vi "Training-Master-Slave.vi"() -> ()   [LabVIEW 2016]
doc: "Use this template to build a master/slave design pattern. The master loop always executes. It notifies one or more slave loops to execute their code. The slave loop(s) continue executing until they complete, then wait for another notification. Contrast this with the Producer/Consumer pattern in which the consumer loops execute only when they have data in their queue."
panel:
  out "notification":dbl[](array[numeric])
  in  "Device":u32
  in  "stop":bool
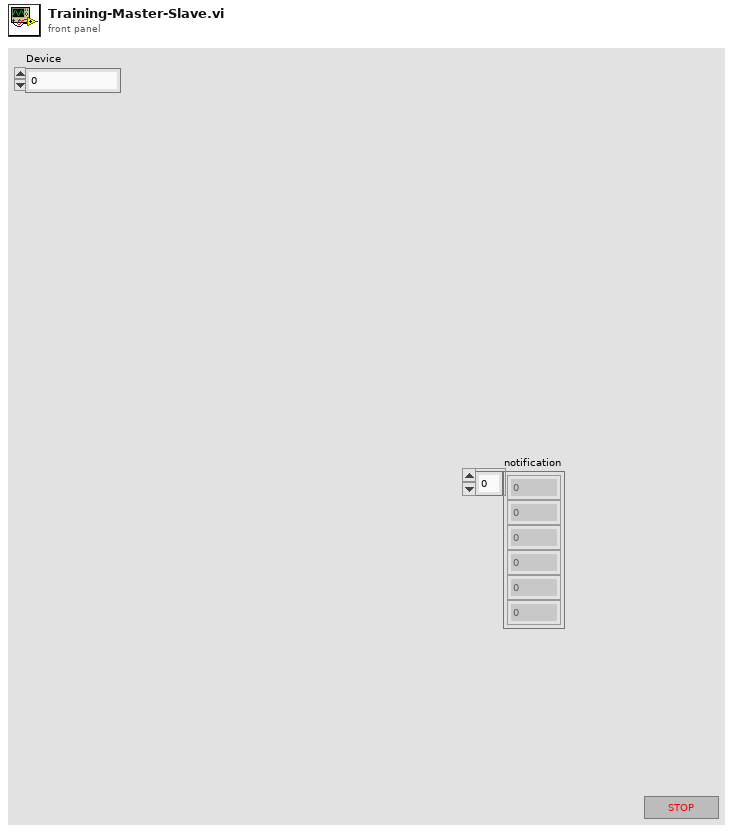
[diagram p1: front panel]
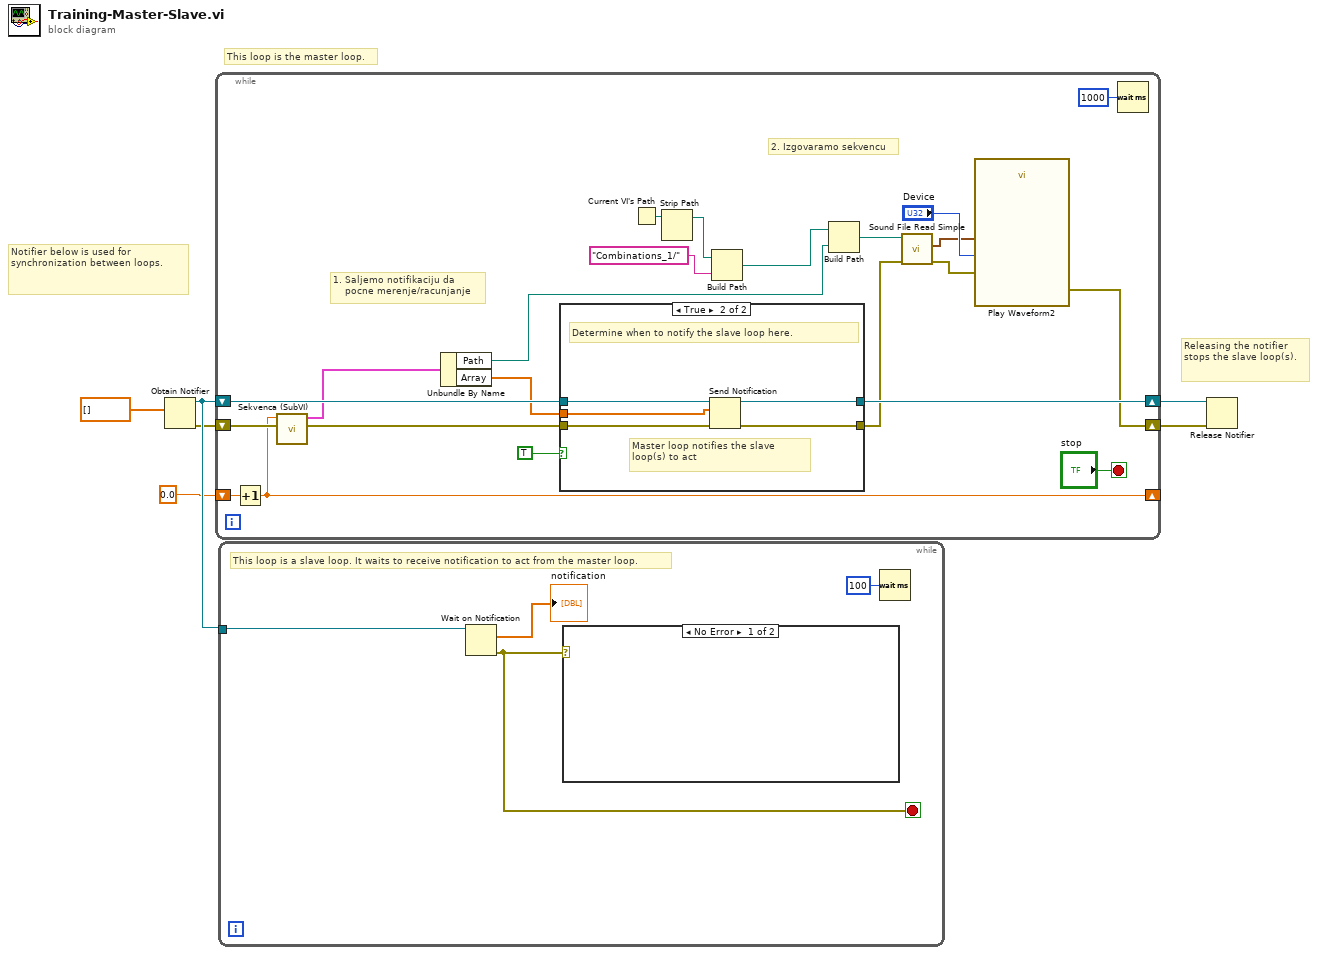
[diagram p0: block diagram]
diagram:
  # "This loop is the master loop."
  # "Releasing the notifier stops the slave loop(s)."
  # "Notifier below is used for  synchronization between loops."
  n1 = Obtain Notifier(notification data type=dbl[] [] ("Array")) -> (notifier out=w6:refnum<notifier>, error out=w5:errorcluster)  [unwired: 2 in, 2 out]
  n2 = while {
    shift-right: [w8] -> w4
    shift-left: w5 -> [w23]
    shift-right: [w25] -> w3
    shift-left: w6 -> [w26]
    shift-right: [w21] -> _
    shift-left: 0.0 -> [w22]
    stop <- "stop" stop-if-true
    # "2. Izgovaramo sekvencu"
    # "1. Saljemo notifikaciju da\n    pocne merenje/racunjanje"
    n3 = Increment(x=w22) -> (x+1=w21:dbl)
    n4 = call "Sekvenca (SubVI).vi"("error in (no error)"=w23, "Ulaz"=w21) -> ("error out"=w10:errorcluster, "Cluster 41"=w20:cluster{"Path":path, "Array":dbl[]})  [unwired: 8 in]
    n5 = Unbundle By Name(w20) -> ("Path"=w12:path, "Array"=w11:dbl[])
    n6 = case shown="True" TRUE ("Case Constant\n(See Context Help)") {
      tunnel: w26 -> [w30 w35]
      tunnel: [w29 w34] -> w9
      tunnel: [w30 w33] -> w25
      tunnel: w10 -> [w29 w32]
      tunnel: w11 -> [_ w31]
      frame False {
      }
      frame True {
        # "Determine when to notify the slave loop here."
        # "Master loop notifies the slave loop(s) to act"
        n7 = Send Notification(notification=w31, notifier=w35, error in (no error)=w32) -> (notifier out=w33:refnum<notifier>, error out=w34:errorcluster)
      }
    }
    n8 = Current VI's Path() -> (path=w17:path)
    n9 = Strip Path(path=w17) -> (stripped path=w14:path)  [unwired: 1 out]
    n10 = Build Path(base path=w14, name or relative path="Combinations_1/") -> (appended path=w16:path)
    n11 = Build Path(base path=w16, name or relative path=w12) -> (appended path=w15:path)
    n12 = call <vilib>:"Sound File Read Simple.vi"("error in (no error)"=w9, "path"=w15) -> ("error out"=w19:errorcluster, "data"=w7:waveform(dbl)[])  [unwired: 6 in, 2 out]
    n13 = call "Play Waveform2"("Device"="Device", "Data"=w7, "error in"=w19) -> ("error out"=w8:errorcluster)  [unwired: 16 in]
    n14 = Wait (ms)(milliseconds to wait=u32 1000) -> ()  [unwired: 1 out]
  }
  n15 = while {
    tunnel: w6 -> [w39]
    stop <- w38 stop-if-true
    # "This loop is a slave loop. It waits to receive notification to act from the master loop."
    n16 = Wait on Notification(notifier=w39) -> (notification=→"notification":dbl[], error out=w38:errorcluster)  [unwired: 1 in, 4 out]
    n17 = case shown="No Error" w38 {
      frame No Error {
      }
      frame Error {
      }
    }
    n18 = Wait (ms)(milliseconds to wait=u32 100) -> ()  [unwired: 1 out]
  }
  n19 = Release Notifier(notifier=w3, error in (no error)=w4) -> ()  [unwired: 4 out]
